vi "SAOMM-QueryFalcon.vi"(0 "PRAMMS-COMM IN":refnum<visa-resource-name>="Hp\u0000\u0002", 2 "Bool Refnum":refnum<vi>, 7 "Signature":u32=1886544237, 11 "Error IN":errorcluster, 13 "CommandCluster":cluster{"Type":string[], "Enum":u32[]}={"Type"=["emtError", "emtAreYouThere", "emtAcknowledgment", "emtGetClientType", "emtClientType", "emtGetImageExposureTime", "emtSetImageExposureTime", "emtImageExposureTime", "emtGetOptimalExposureTime", "emtSetOptimalExposureTime", "emtOptimalExposureTime", "emtGetImageEMGain", "emtSetImageEMGain", "emtImageEMGain", "emtGetFPGACtrl", "emtSetFPGACtrl", "emtFPGACtrl", "emtGetImageWidth", "emtSetImageWidth", "emtImageWidth", "emtGetImageHeight", "emtSetImageHeight", "emtImageHeight", "emtGetImageBinning", "emtSetImageBinning", "emtImageBinning", "emtGetImageDisplayFrameRate", "emtSetImageDisplayFrameRate", "emtImageDisplayFrameRate", "emtGetROIWidth", "emtSetROIWidth", "emtROIWidth", "emtGetROIHeight", "emtSetROIHeight", "emtROIHeight", "emtGetROIXOffset", "emtSetROIXOffset", "emtROIXOffset", "emtGetROIYOffset", "emtSetROIYOffset", "emtROIYOffset", "emtStartAcquisition", "mtStopAcquisition", "emtAcquisitionStarted", "emtAcquisitionStopped", "emtGetFalconImage", "emtFalconImage"], "Enum"=[1, 2, 3, 4, 5, 1001, 1101, 1201, 1002, 1102, 1202, 1003, 1103, 1203, 1004, 1104, 1204, 1005, 1105, 1205, 1006, 1106, 1206, 1007, 1107, 1207, 1008, 1108, 1208, 1009, 1109, 1209, 1010, 1110, 1210, 1011, 1111, 1211, 1012, 1112, 1212, 1130, 1131, 1150, 1151, 1070, 1270]}) -> (4 "PRAMMS-COMM OUT":refnum<visa-resource-name>, 15 "Error OUT":errorcluster)   [LabVIEW 2019]
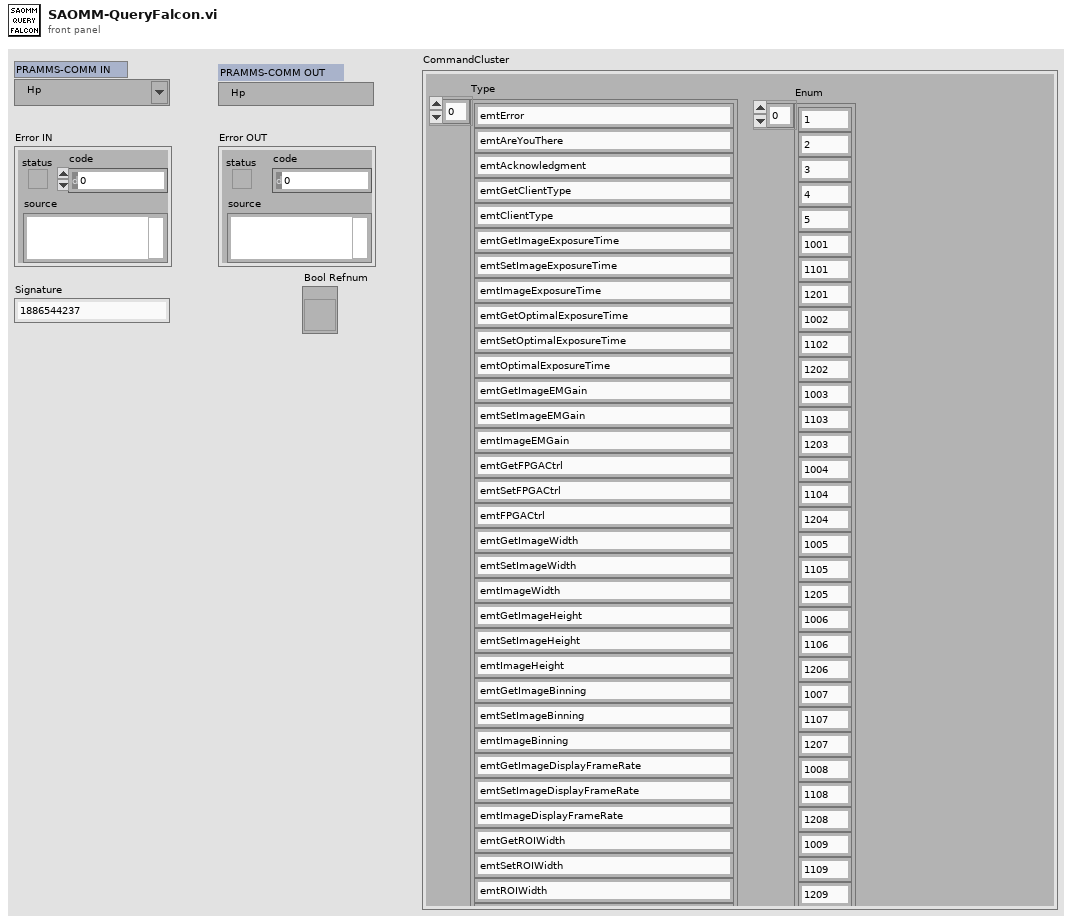
[diagram p1: front panel]
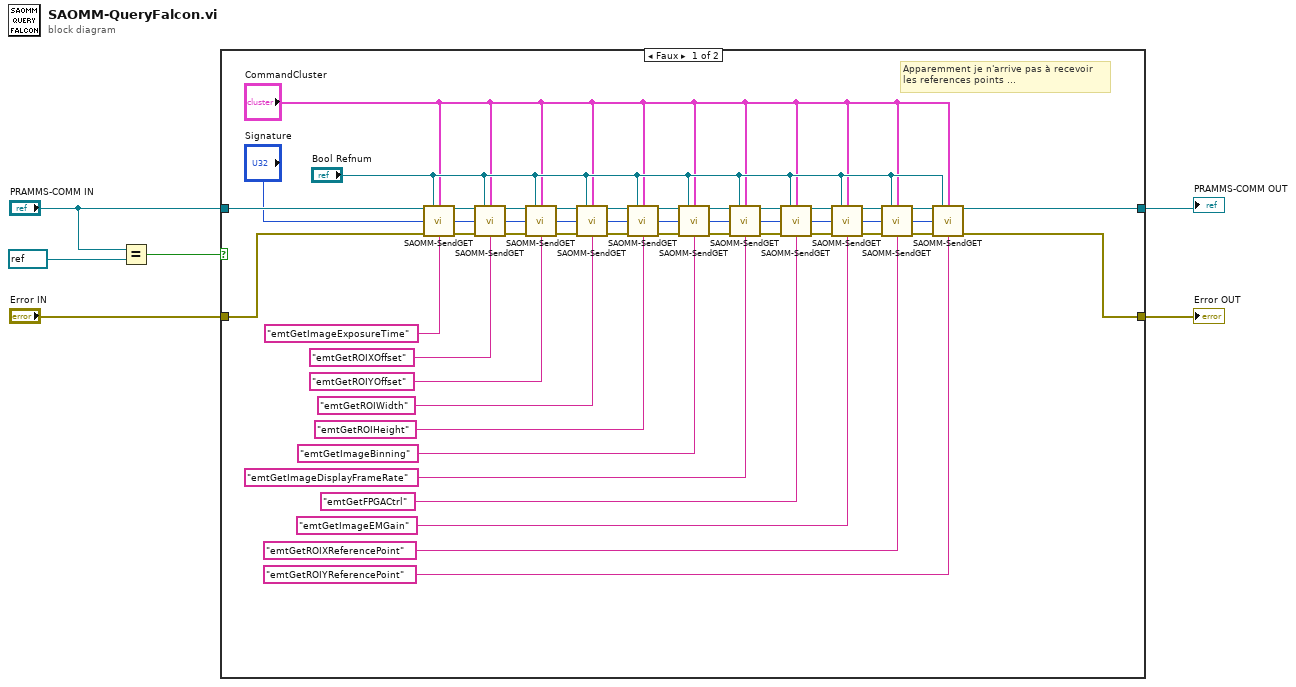
[diagram p0: block diagram]
diagram:
  n1 = Equal?(x="PRAMMS-COMM IN", y=refnum<visa-resource-name> "-1") -> (x = y?=w3:bool)
  n2 = case shown="Faux" w3 {
    tunnel: [w9 w46] -> w6
    tunnel: "PRAMMS-COMM IN" -> [w32 w46]
    tunnel: "Error IN" -> [w33 w45]
    tunnel: [w10 w45] -> w1
    frame False {
      # "Apparemment je n'arrive pas à recevoir\nles references points ..."
      n3 = call "SAOMM-SendGET.vi"("PRAMMS-COMM IN"=w32, "Bool Refnum"="Bool Refnum", "MessageType"="CommandCluster", "Signature"="Signature", "Error IN"=w33, "Active GET"="emtGetImageExposureTime") -> ("PRAMMS-COMM OUT"=w22:refnum<visa-resource-name>, "Error OUT"=w21:errorcluster)  [unwired: 8 in]
      n4 = call "SAOMM-SendGET.vi"("PRAMMS-COMM IN"=w22, "Bool Refnum"="Bool Refnum", "MessageType"="CommandCluster", "Signature"="Signature", "Error IN"=w21, "Active GET"="emtGetROIXOffset") -> ("PRAMMS-COMM OUT"=w41:refnum<visa-resource-name>, "Error OUT"=w39:errorcluster)  [unwired: 8 in]
      n5 = call "SAOMM-SendGET.vi"("PRAMMS-COMM IN"=w41, "Bool Refnum"="Bool Refnum", "MessageType"="CommandCluster", "Signature"="Signature", "Error IN"=w39, "Active GET"="emtGetROIYOffset") -> ("PRAMMS-COMM OUT"=w40:refnum<visa-resource-name>, "Error OUT"=w38:errorcluster)  [unwired: 8 in]
      n6 = call "SAOMM-SendGET.vi"("PRAMMS-COMM IN"=w40, "Bool Refnum"="Bool Refnum", "MessageType"="CommandCluster", "Signature"="Signature", "Error IN"=w38, "Active GET"="emtGetROIWidth") -> ("PRAMMS-COMM OUT"=w36:refnum<visa-resource-name>, "Error OUT"=w35:errorcluster)  [unwired: 8 in]
      n7 = call "SAOMM-SendGET.vi"("PRAMMS-COMM IN"=w36, "Bool Refnum"="Bool Refnum", "MessageType"="CommandCluster", "Signature"="Signature", "Error IN"=w35, "Active GET"="emtGetROIHeight") -> ("PRAMMS-COMM OUT"=w31:refnum<visa-resource-name>, "Error OUT"=w30:errorcluster)  [unwired: 8 in]
      n8 = call "SAOMM-SendGET.vi"("PRAMMS-COMM IN"=w31, "Bool Refnum"="Bool Refnum", "MessageType"="CommandCluster", "Signature"="Signature", "Error IN"=w30, "Active GET"="emtGetImageBinning") -> ("PRAMMS-COMM OUT"=w29:refnum<visa-resource-name>, "Error OUT"=w28:errorcluster)  [unwired: 8 in]
      n9 = call "SAOMM-SendGET.vi"("PRAMMS-COMM IN"=w29, "Bool Refnum"="Bool Refnum", "MessageType"="CommandCluster", "Signature"="Signature", "Error IN"=w28, "Active GET"="emtGetImageDisplayFrameRate") -> ("PRAMMS-COMM OUT"=w25:refnum<visa-resource-name>, "Error OUT"=w24:errorcluster)  [unwired: 8 in]
      n10 = call "SAOMM-SendGET.vi"("PRAMMS-COMM IN"=w25, "Bool Refnum"="Bool Refnum", "MessageType"="CommandCluster", "Signature"="Signature", "Error IN"=w24, "Active GET"="emtGetFPGACtrl") -> ("PRAMMS-COMM OUT"=w20:refnum<visa-resource-name>, "Error OUT"=w19:errorcluster)  [unwired: 8 in]
      n11 = call "SAOMM-SendGET.vi"("PRAMMS-COMM IN"=w20, "Bool Refnum"="Bool Refnum", "MessageType"="CommandCluster", "Signature"="Signature", "Error IN"=w19, "Active GET"="emtGetImageEMGain") -> ("PRAMMS-COMM OUT"=w17:refnum<visa-resource-name>, "Error OUT"=w16:errorcluster)  [unwired: 8 in]
      n12 = call "SAOMM-SendGET.vi"("PRAMMS-COMM IN"=w17, "Bool Refnum"="Bool Refnum", "MessageType"="CommandCluster", "Signature"="Signature", "Error IN"=w16, "Active GET"="emtGetROIXReferencePoint") -> ("PRAMMS-COMM OUT"=w8:refnum<visa-resource-name>, "Error OUT"=w7:errorcluster)  [unwired: 8 in]
      n13 = call "SAOMM-SendGET.vi"("PRAMMS-COMM IN"=w8, "Bool Refnum"="Bool Refnum", "MessageType"="CommandCluster", "Signature"="Signature", "Error IN"=w7, "Active GET"="emtGetROIYReferencePoint") -> ("PRAMMS-COMM OUT"=w9:refnum<visa-resource-name>, "Error OUT"=w10:errorcluster)  [unwired: 8 in]
    }
    frame True {
    }
  }
  "PRAMMS-COMM OUT" <- w6
  "Error OUT" <- w1
